vi "Drive Controller.vi"(8 "error in":errorcluster) -> ()   [LabVIEW 2016]
doc: "This VI executes continuously carrying out the current operation and responding to updates or new operation requests. It will often contain the timing or control code that is difficult to place directly in TeleOp. This VI generally opens all sensors and motors and isolates the rest of the robot code from knowing implementation details of how the operations are carried out."
uses:
  Drive Setpoints.ctl
  Drive Operations.ctl
  <vilib>/Rock Robotics/WPI/SafetyOutput/WPI_SafetyOutputConfigMenu.ctl
  <vilib>/Rock Robotics/WPI/ThirdParty/CanMotor/TalonSRX/WPI_CANTalonSRX_APIControlMode.ctl
  <vilib>/Rock Robotics/WPI/ThirdParty/CanMotor/TalonSRX/WPI_CANTalonSRX_APIFeedbackSelect.ctl
  <vilib>/Rock Robotics/WPI/Solenoid/WPI_SolenoidValue.ctl
  <vilib>/Rock Robotics/WPI/RobotDrive/WPI_RobotDriveOpen2MotorWithExistingMotors.vi
  Framework/Robot Global Data.vi
  <vilib>/Rock Robotics/Network Tables/NT Write Number.vi
  <vilib>/Rock Robotics/Network Tables/NT Write String.vi
  <vilib>/Rock Robotics/WPI/Solenoid/WPI_SolenoidGetEnum.vi
panel:
  in  "Front View":bool
  out "Setpoints":T1(graph)
  out "Current\nCmd":string
  # "Tip: It may be helpful to observe inputs and sensor values.\nYou may also want to display tuning or debugging controls."
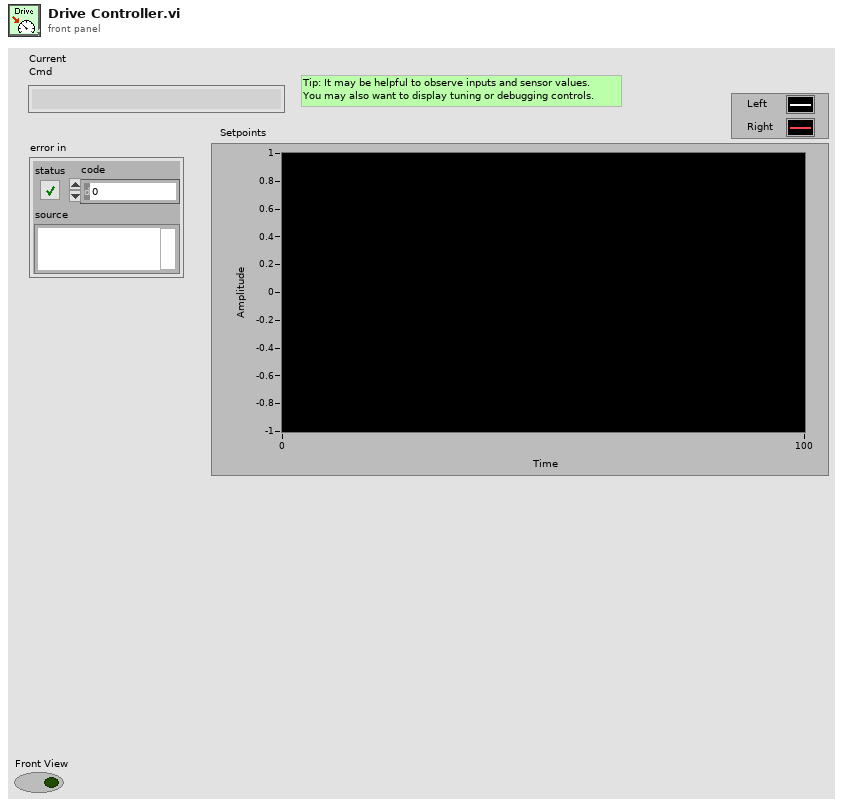
[diagram p1: front panel]
types:
  T1 = cluster{"Left Setpoint":dbl, "Right Setpoint":dbl}
  T2 = typedef "WPI_CANTalonSRX_APIFeedbackSelect.ctl" = enum16{"Digital Quadrature Encoder", "Analog Potentiometer", "Analog Encoder", "Count on Quad-A (Rising-Edge)", "Count on Quad-A (Falling-Edge)", "CTR Magnetic Enc (Absolute)", "CTR Magnetic Enc (Relative)", "Pulse Width"}
  T3 = typedef "WPI_CANTalonSRX_APIControlMode.ctl" = enum8{"Percent VBus", "Speed", "Position", "Slave", "Unchanged / Invalid", "Voltage Compensation", "Current", "Motion Profile", "Motion Magic"}
  T4 = typedef "WPI_SafetyOutputConfigMenu.ctl" = enum16{"Enable", "Disable"}
  T5 = typedef "Drive Setpoints.ctl" = cluster{"Operation":T6, "Left Setpoint":dbl, "Right Setpoint":dbl, "Duration":dbl}
  T6 = typedef "Drive Operations.ctl" = enum16{"Reserve", "Read Current", "Immediate", "Drive for Time", "Drive for Distance", "Drive for Angle"}
  T7 = typedef "WPI_MotorControlDeviceRef.ctl" = cluster{"DeviceStatus":errorcluster, "Type":T8, "PWM":cluster{"PWM Channel":T9, "DeadBand":T10}, "CAN":cluster{"Device Number":u8, "SetOutput VI Ref":variant, "GetOutput VI Ref":variant, "Enable VI Ref":variant, "Disable VI Ref":variant, "Data":variant}, "Invert":bool}
  T8 = typedef "WPI_MotorControlType.ctl" = enum16{"PWM", "CAN"}
  T9 = typedef "FPGA_DIOPWMChannel.ctl" = enum8{"PWM 0", "PWM 1", "PWM 2", "PWM 3", "PWM 4", "PWM 5", "PWM 6", "PWM 7", "PWM 8", "PWM 9", "PWM MXP 0", "PWM MXP 1", "PWM MXP 2", "PWM MXP 3", "PWM MXP 4", "PWM MXP 5", "PWM MXP 6", "PWM MXP 7", "PWM MXP 8", "PWM MXP 9", "Invalid"}
  T10 = typedef "WPI_PWMDeadband.ctl" = cluster{"Name":string, "maxPositivePwm":i32, "minPositivePwm":i32, "centerPwm":i32, "maxNegativePwm":i32, "minNegativePwm":i32, "angularRange":u16}
  T11 = typedef "WPI_RobotDriveDevRef.ctl" = cluster{"DevStatus":errorcluster, "Motors[]":T7[], "Square Inputs":bool, "Max Output":dbl}
  T12 = typedef "Command Status Info.ctl" = cluster{"Name":string, "Status":T13, "notifier out":T14}
  T13 = typedef "Completion Status.ctl" = enum16{"Successful", "Aborted", "Incomplete"}
  T14 = typedef "Completion Notifier.ctl" = refnum<notifier>
  T15 = cluster{"SubSystem Data":T5, cluster{"Start Time (ms)":u32, "Iterations":i32}, cluster{"Command Info":T12, "Description":string, "SubSystem Data":T5, "notifier out":refnum<notifier>, "Subsystem Name":string}}
  T16 = typedef "WPI_SolenoidValue.ctl" = enum16{"Off", "On", "Forward", "Reverse"}
  T17 = typedef "WPI_SolenoidDevRef.ctl" = cluster{"DevStatus":errorcluster, "Pneumatics Control Module":u8, "Forward Solenoid Channel":T18, "Reverse Solenoid Channel":T18}
  T18 = typedef "WPI_SolenoidChannel.ctl" = enum8{"Solenoid 0", "Solenoid 1", "Solenoid 2", "Solenoid 3", "Solenoid 4", "Solenoid 5", "Solenoid 6", "Solenoid 7", "Invalid"}
  T19 = cluster{"SubSystem Data":T5, cluster{"Start Time (ms)":u32, "Iterations":i32}, "Default Command Arguments":cluster{"Command Info":T12, "Description":string, "SubSystem Data":T5, "notifier out":refnum<notifier>, "Subsystem Name":string}}
  T20 = typedef "WPI_CANTalonSRX_GlobalStatus.ctl" = cluster{"Applied Throttle":dbl, "Module Enabled":bool, "CAN Error":errorcluster, "Closed Loop Error":dbl, "Forward Limit Switch Closed":bool, "Reverse Limit Switch Closed":bool, "Sensor Position":dbl, "Sensor Velocity":dbl, "Current":dbl, "Sticky Fault - Over Temp":bool, "Sticky Fault - Under Voltage":bool, "Sticky Fault - Forward Limit":bool, "Sticky Fault - Reverse Limit":bool, "Sticky Fault - Forward Soft Limit":bool, "Sticky Fault - Reverse Soft Limit":bool, "Brake is Enabled":bool, "Encoder Position":dbl, "Encoder Velocity":dbl, "Encoder Index Count":dbl, "Encoder A Pin State":bool, "Encoder B Pin State":bool, "Encoder Index Pin State":bool, "Analog In":dbl, "Analog In Velocity":dbl, "Temperature (C)":dbl, "Battery Voltage":dbl, "Control 5 Is Supported":bool, "Current Profile Slot Select":dbl, "Pos Div 8":bool, "Vel Div 4":bool, "Pulse Width Position":i32, "Pulse Width Velocity":i32, "Pulse Width Rise To Rise (us)":i32, "Pulse Width Rise To Fall (us)":i32, "Mot Prof Active Is Under Run":bool, "Mot Prof Active Has Under Run":bool, "Mot Prof Active Is Last":bool, "Mot Prof Active Velocity Only":bool, "Mot Prof Active Is Valid":bool, "Mot Prof Buffer Is Full":bool, "Mot Prof Active Profile Slot Select":i32, "Mot Prof NextID":i32, "Mot Prof Count":i32, "Mot Prof Active Velocity":dbl, "Mot Prof Active Position":dbl, "Mot Prof Output Enable":i32}
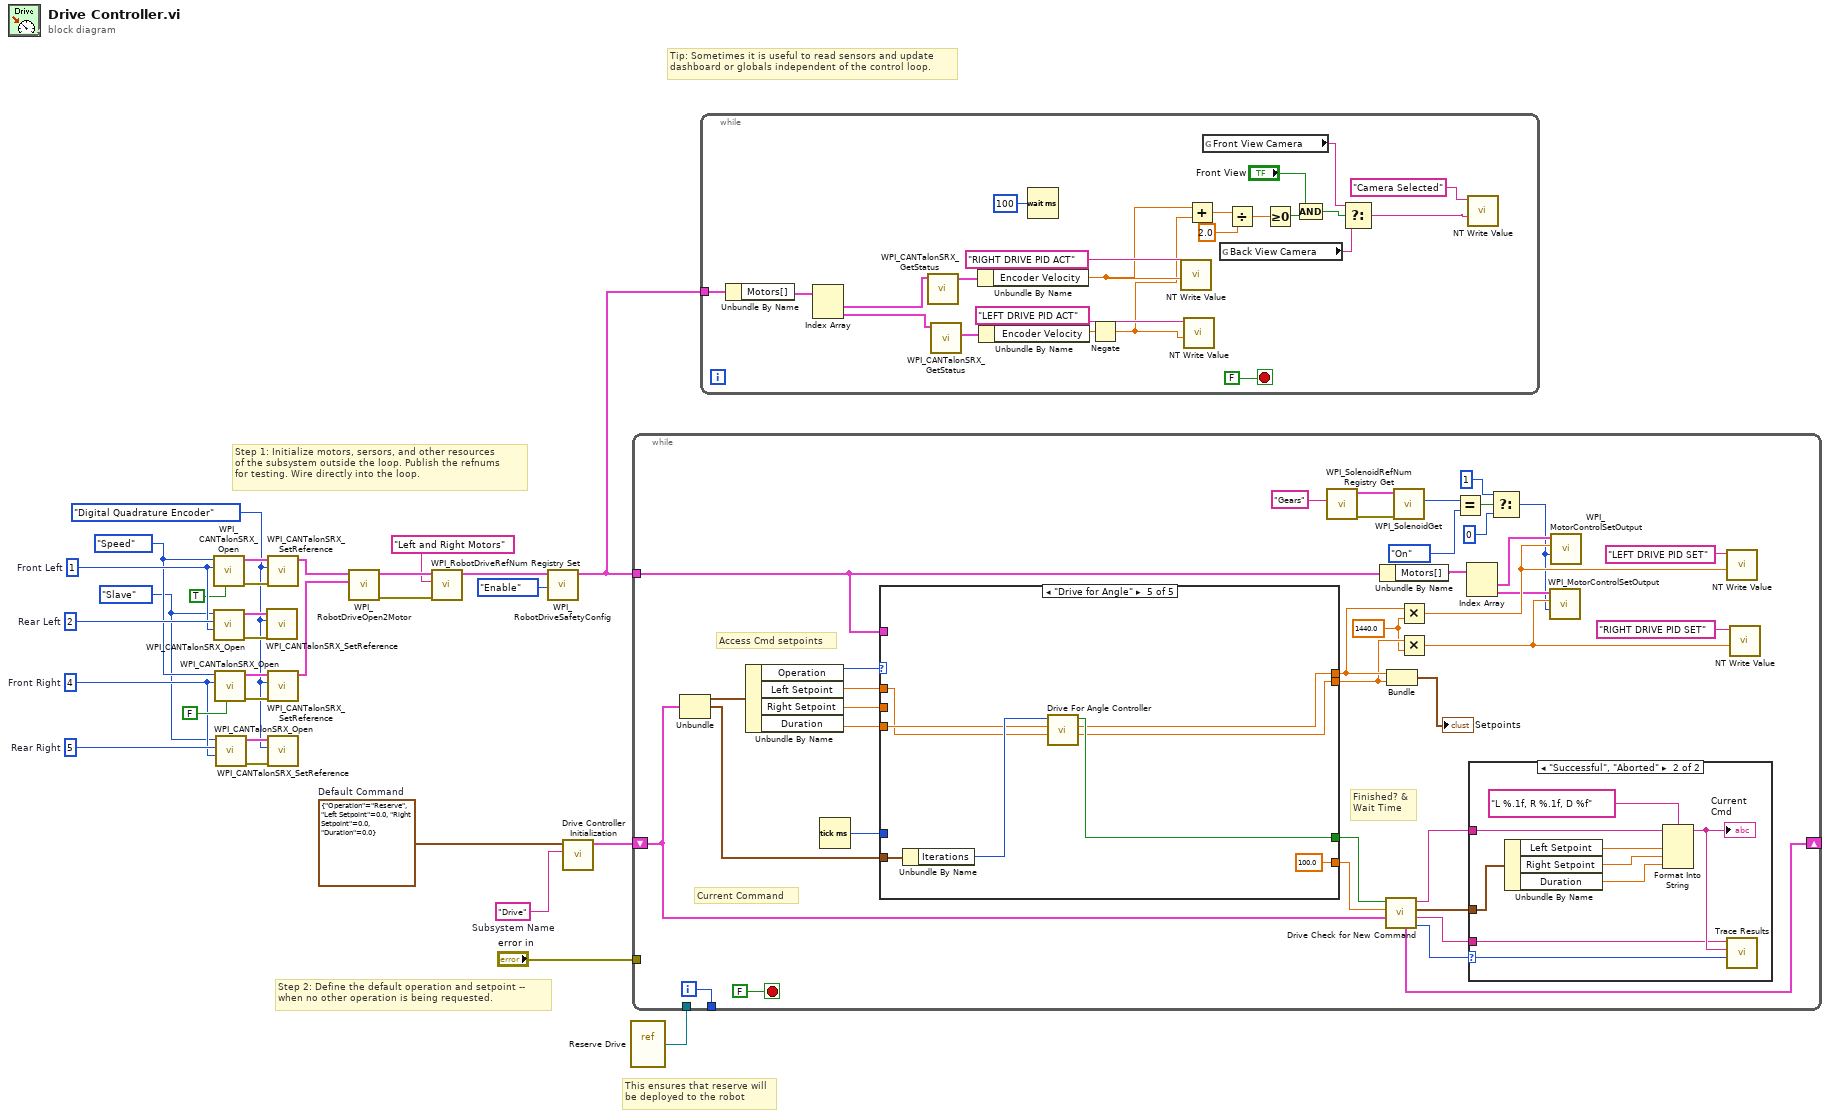
[diagram p0: block diagram]
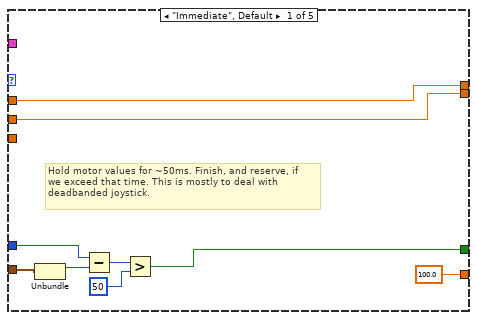
[diagram p3: hidden frame]
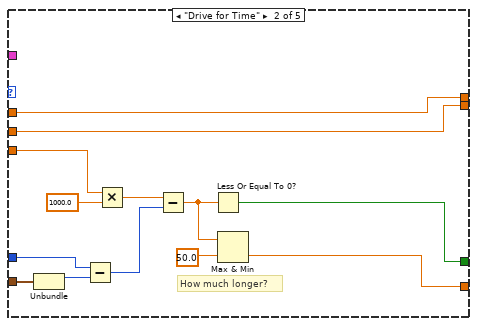
[diagram p4: hidden frame]
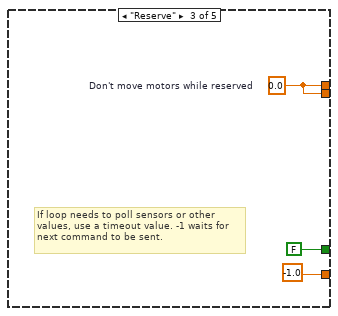
[diagram p5: hidden frame]
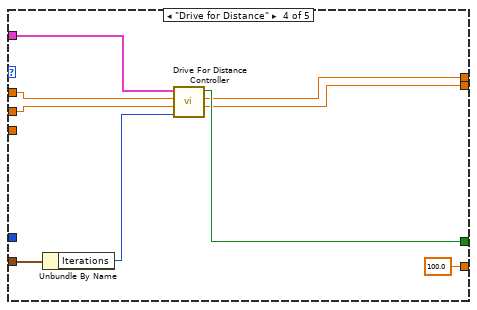
[diagram p6: hidden frame]
diagram:
  w1 = WPI_CANTalonSRX_APIFeedbackSelect."Digital Quadrature Encoder" ("Feedback Reference")
  w13 = WPI_CANTalonSRX_APIControlMode."Slave" ("Control Mode")
  w14 = WPI_CANTalonSRX_APIControlMode."Speed" ("Control Mode")
  w16 = 5  # Rear Right
  w15 = 4  # Front Right
  w18 = 2  # Rear Left
  w17 = 1  # Front Left
  w29 = T5 {"Operation"=enum."Reserve", "Left Setpoint"=0.0, "Right Setpoint"=0.0, "Duration"=0.0}  # Default Command
  w30 = "Drive"  # Subsystem Name
  # "This ensures that reserve will\nbe deployed to the robot"
  # "Tip: Sometimes it is useful to read sensors and update\ndashboard or globals independent of the control loop."
  # "Step 2: Define the default operation and setpoint --\nwhen no other operation is being requested."
  # "Step 1: Initialize motors, sersors, and other resources\nof the subsystem outside the loop. Publish the refnums\nfor testing. Wire directly into the loop."
  n1 = call <vilib>:"WPI_CANTalonSRX_Open.vi"("Invert"=TRUE, "Device Number"=w17, "Control Mode"=w14) -> ("error out"=w7:errorcluster, "CAN Talon SRX Ref"=w6:T7)  [unwired: 7 in]
  n2 = call <vilib>:"WPI_CANTalonSRX_Open.vi"("Master Device Number"=w17, "Device Number"=w18, "Control Mode"=w13) -> ("error out"=w9:errorcluster, "CAN Talon SRX Ref"=w8:T7)  [unwired: 7 in]
  n3 = call <vilib>:"WPI_CANTalonSRX_Open.vi"("Invert"=FALSE, "Device Number"=w15, "Control Mode"=w14) -> ("error out"=w4:errorcluster, "CAN Talon SRX Ref"=w3:T7)  [unwired: 7 in]
  n4 = call <vilib>:"WPI_CANTalonSRX_Open.vi"("Master Device Number"=w15, "Device Number"=w16, "Control Mode"=w13) -> ("error out"=w11:errorcluster, "CAN Talon SRX Ref"=w10:T7)  [unwired: 7 in]
  n5 = call <vilib>:"WPI_CANTalonSRX_SetReference.vi"("error in (no error)"=w9, "Feedback Reference"=w1, "CAN Talon SRX Ref"=w8) -> ()  [unwired: 7 in, 2 out]
  n6 = call <vilib>:"WPI_CANTalonSRX_SetReference.vi"("error in (no error)"=w7, "Feedback Reference"=w1, "CAN Talon SRX Ref"=w6) -> ("CAN Talon SRX Ref"=w5:T7)  [unwired: 7 in, 1 out]
  n7 = call <vilib>:"WPI_CANTalonSRX_SetReference.vi"("error in (no error)"=w4, "Feedback Reference"=w1, "CAN Talon SRX Ref"=w3) -> ("CAN Talon SRX Ref"=w2:T7)  [unwired: 7 in, 1 out]
  n8 = call <vilib>:"WPI_CANTalonSRX_SetReference.vi"("error in (no error)"=w11, "Feedback Reference"=w1, "CAN Talon SRX Ref"=w10) -> ()  [unwired: 7 in, 2 out]
  n9 = call-poly <vilib>:"WPI_RobotDriveOpen2Motor.vi"("Right Motor Dev Ref"=w2, "Left Motor Dev Ref"=w5) -> ("error out"=w26:errorcluster, "RobotDriveDevRef"=w28:T11)  [unwired: 3 in, 5 out]
  n10 = call <vilib>:"WPI_RobotDriveRefNum Registry Set.vi"("error in (no error)"=w26, "refnum name"="Left and Right Motors", "RobotDriveDevRef"=w28) -> ("RobotDriveDevRef"=w25:T11)  [unwired: 1 in, 7 out]
  n11 = call <vilib>:"WPI_RobotDriveSafetyConfig.vi"("mode"=WPI_SafetyOutputConfigMenu."Enable", "RobotDriveDevRef"=w25) -> ("RobotDriveDevRef"=w23:T11)  [unwired: 8 in, 1 out]
  n12 = call "Drive Controller Initialization.vi"("Subsystem Name"=w30, "Default Command"=w29) -> ("output cluster"=w21:T15)  [unwired: 9 in]
  n13 = vi-ref "Reserve Drive.vi"() -> (w20:refnum<vi>)
  n14 = while {
    shift-right: [w58] -> _
    shift-left: w21 -> [w51]
    tunnel: [w67] -> _
    tunnel: w23 -> [w43]
    tunnel: "error in" -> [_]
    tunnel: w20 -> [_]
    i -> [w67]
    stop <- FALSE stop-if-true
    w48 = 1440.0 ("y")
    # "Current Command"
    # "Access Cmd setpoints"
    # "Finished? &\nWait Time"
    n15 = Unbundle(w51) -> ("SubSystem Data"=w65:T5, w52:cluster{"Start Time (ms)":u32, "Iterations":i32})  [unwired: 1 out]
    n16 = Unbundle By Name(w65) -> ("Operation"=w64:T6, "Left Setpoint"=w63:dbl, "Right Setpoint"=w62:dbl, "Duration"=w61:dbl)
    n17 = Tick Count (ms)() -> (millisecond timer value=w60:u32)
    n18 = case shown="\"Drive for Angle\"" w64 {
      tunnel: [100.0 w87 -1.0 100.0 100.0] -> w57
      tunnel: [w79 w94 FALSE ("ignore previous (F)") w107 w115] -> w56
      tunnel: w52 -> [w78 w96 _ w110 w119]
      tunnel: [w85 w93 w100 w105 w113] -> w50
      tunnel: [w84 w92 w100 w104 w112] -> w49
      tunnel: w63 -> [w85 w93 _ w109 w116]
      tunnel: w62 -> [w84 w92 _ w108 _]
      tunnel: w61 -> [_ w91 _ _ w117]
      tunnel: w60 -> [w80 w90 _ _ _]
      tunnel: w43 -> [_ _ _ w111 _]
      frame "Immediate", Default {
        # "Hold motor values for ~50ms. Finish, and reserve, if\nwe exceed that time. This is mostly to deal with\ndeadbanded joystick."
        n19 = Unbundle(w78) -> ("Start Time (ms)"=w81:u32)  [unwired: 1 out]
        n20 = Subtract(x=w80, y=w81) -> (x-y=w82:u32)
        n21 = Greater?(x=w82, y=u8 50 ("Left Motor")) -> (0:w79:bool)
      }
      frame "Drive for Time" {
        # "How much longer?"
        n22 = Unbundle(w96) -> ("Start Time (ms)"=w95:u32)  [unwired: 1 out]
        n23 = Subtract(x=w90, y=w95) -> (x-y=w99:u32)
        n24 = Multiply(x=w91, y=1000.0) -> (x*y=w98:dbl)
        n25 = Subtract(x=w98, y=w99) -> (x-y=w89:dbl)
        n26 = Less Or Equal To 0?(x=w89) -> (x <= 0?=w94:bool)
        n27 = Max & Min(x=w89, y=50.0) -> (min(x,y)=w87:dbl)  [unwired: 1 out]
      }
      frame "Reserve" {
        w100 = 0.0  # Don't move motors while reserved
        # "If loop needs to poll sensors or other\nvalues, use a timeout value. -1 waits for\nnext command to be sent."
      }
      frame "Drive for Distance" {
        n28 = Unbundle By Name(w110) -> ("Iterations"=w103:i32)
        n29 = call "Drive For Distance Controller.vi"("Command Iteration"=w103, "Speed"=w108, "Distance (in)"=w109, "RobotDriveDevRef"=w111) -> ("Right Setpoint"=w104:dbl, "Left Setpoint"=w105:dbl, "Finished?"=w107:bool)  [unwired: 5 in]
      }
      frame "Drive for Angle" {
        n30 = Unbundle By Name(w119) -> ("Iterations"=w118:i32)
        n31 = call "Drive For Angle Controller.vi"("Speed"=w116, "Yaw"=w117, "Iterations"=w118) -> ("Right Setpoint"=w112:dbl, "Left Setpoint"=w113:dbl, "Finished?"=w115:bool)  [unwired: 6 in]
      }
    }
    n32 = call <vilib>:"WPI_SolenoidRefNum Registry Get.vi"("refnum name"="Gears") -> ("error out"=w39:errorcluster, "SolenoidDevRef"=w40:T17)  [unwired: 9 in]
    n33 = Unbundle By Name(w43) -> ("Motors[]"=w44:T7[])
    n34 = call "Drive Check for New Command.vi"("input cluster"=w51, "Wait time (ms)"=w57, "Finished?"=w56) -> ("Completion"=w59:T13, "Subsystem Name"=w53:string, "SetPoint"=w54:T5, "Initial Trace String"=w55:string, "output cluster"=w58:T19)  [unwired: 4 in]
    n35 = Bundle("Left Setpoint"=w50, "Right Setpoint"=w49) -> (→"Setpoints":T1)  [unwired: 1 in]
    n36 = call-poly <vilib>:"WPI_SolenoidGet.vi"("error in (no error)"=w39, "SolenoidDevRef"=w40) -> ("Value"=w38:T16)  [unwired: 7 in, 2 out]
    n37 = Multiply(x=w50, y=w48) -> (x*y=w41:dbl)
    n38 = Multiply(x=w49, y=w48) -> (x*y=w32:dbl)
    n39 = Equal?(x=w38, y=WPI_SolenoidValue."On" ("Value")) -> (x = y?=w36:bool)
    n40 = Index Array(array=w44) -> (element #1=w42:T7, element #2=w33:T7)  [unwired: 2 in]
    n41 = case shown="\"Successful\", \"Aborted\"" w59 {
      selector: w59 -> [_ w77]
      tunnel: w55 -> [_ w72]
      tunnel: w54 -> [_ w73]
      tunnel: w53 -> [_ w69]
      frame "Incomplete", Default {
        # "Continuing current command"
      }
      frame "Successful", "Aborted" {
        # "Report and setup for next command"
        n42 = Unbundle By Name(w73) -> ("Left Setpoint"=w75:dbl, "Right Setpoint"=w76:dbl, "Duration"=w70:dbl)
        n43 = Format Into String(format string="L %.1f, R %.1f, D %f", initial string=w72, w75, w76, w70) -> (resulting string=w71:string)  [unwired: 1 in, 1 out]
        "Current\nCmd" <- w71
        n44 = call <vilib>:"Trace Results.vi"("Status of previous command"=w77, "Description"=w71, "Subsystem"=w69) -> ()  [unwired: 9 in]
      }
    }
    n45 = Select(t=1, s=w36, f=0 ("t")) -> (s? t:f=w31:i32)
    n46 = call <vilib>:"WPI_MotorControlSetOutput.vi"("options"=w31, "Output"=w32, "MotorControlDevRef"=w33) -> ()  [unwired: 6 in, 3 out]
    n47 = call <vilib>:"WPI_MotorControlSetOutput.vi"("options"=w31, "Output"=w41, "MotorControlDevRef"=w42) -> ()  [unwired: 6 in, 3 out]
    n48 = call-poly <vilib>:"NT Write Value.vi"("Numeric"=w41, "Name"="LEFT DRIVE PID SET") -> ()  [unwired: 9 in, 1 out]
    n49 = call-poly <vilib>:"NT Write Value.vi"("Numeric"=w32, "Name"="RIGHT DRIVE PID SET") -> ()  [unwired: 9 in, 1 out]
  }
  n50 = while {
    tunnel: w23 -> [w140]
    stop <- FALSE stop-if-true
    n51 = Unbundle By Name(w140) -> ("Motors[]"=w139:T7[])
    n52 = Index Array(array=w139) -> (element #1=w136:T7, element #2=w135:T7)  [unwired: 2 in]
    n53 = call <vilib>:"WPI_CANTalonSRX_GetStatus.vi"("CAN Talon SRX Ref"=w136) -> ("Talon SRX Status"=w134:T20)  [unwired: 8 in, 2 out]
    n54 = call <vilib>:"WPI_CANTalonSRX_GetStatus.vi"("CAN Talon SRX Ref"=w135) -> ("Talon SRX Status"=w133:T20)  [unwired: 8 in, 2 out]
    n55 = Unbundle By Name(w134) -> ("Encoder Velocity"=w131:dbl)
    n56 = Unbundle By Name(w133) -> ("Encoder Velocity"=w132:dbl)
    n57 = Wait (ms)(milliseconds to wait=u32 100) -> ()  [unwired: 1 out]
    n58 = Negate(x=w132) -> (-x=w130:dbl)
    n59 = call-poly <vilib>:"NT Write Value.vi"("Numeric"=w131, "Name"="RIGHT DRIVE PID ACT") -> ()  [unwired: 9 in, 1 out]
    n60 = call-poly <vilib>:"NT Write Value.vi"("Numeric"=w130, "Name"="LEFT DRIVE PID ACT") -> ()  [unwired: 9 in, 1 out]
    n61 = Add(x=w131, y=w130) -> (x+y=w129:dbl)
    n62 = global read "Robot Global Data.vi" "Front View Camera"() -> (w124:string)
    n63 = global read "Robot Global Data.vi" "Back View Camera"() -> (w123:string)
    n64 = Divide(x=w129, y=2.0) -> (x/y=w126:dbl)
    n65 = Greater Or Equal To 0?(x=w126) -> (x >= 0?=w122:bool)
    n66 = Compound Arithmetic op=AND("Front View", w122) -> (w121:bool)
    n67 = Select(t=w124, s=w121, f=w123) -> (s? t:f=w125:string)
    n68 = call-poly <vilib>:"NT Write Value.vi"("String"=w125, "Name"="Camera Selected") -> ()  [unwired: 9 in, 1 out]
  }
